vi "Get Variables.vi"(8 "error in (no error)":errorcluster, 11 "functionbase in":refnum<class "functionbase.lvclass">) -> (0 "error out":errorcluster, 2 "Variables":variant, 3 "functionbase out":refnum<class "functionbase.lvclass">)   [LabVIEW 2019, in "LSL.lvlib" / "functionbase.lvclass"]
uses:
  functionbase.lvclass
  typedefs/Variables.ctl
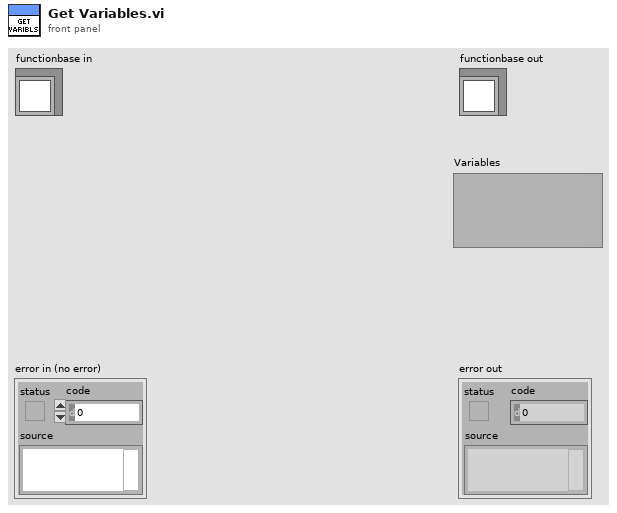
[diagram p1: front panel]
types:
  T1 = typedef "LSL.lvlib/functionbase.lvclass/Variables.ctl" = cluster{"BoringEngineer":string}
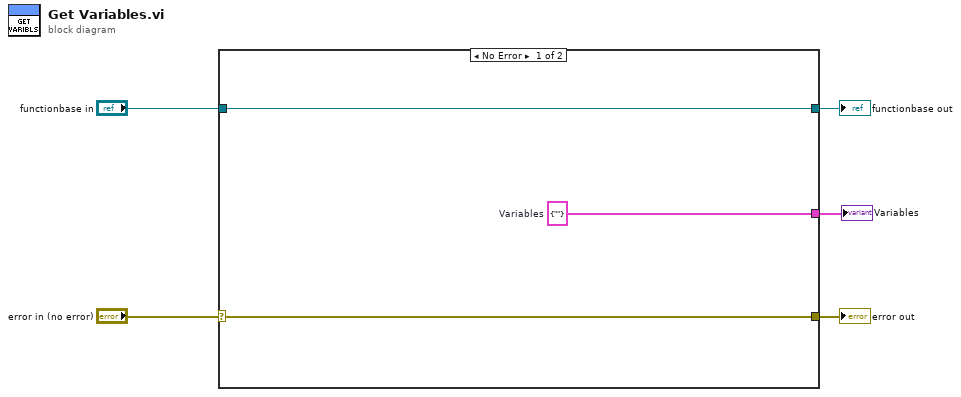
[diagram p0: block diagram]
diagram:
  n1 = case shown="No Error" "error in (no error)" {
    selector: "error in (no error)" -> [w8 w10]
    tunnel: [w8 w10] -> w4
    tunnel: [w7 w9] -> w2
    tunnel: "functionbase in" -> [w7 w9]
    tunnel: [w6 _] -> w1
    frame No Error {
      w6 = T1 {"BoringEngineer"=""}  # Variables
    }
    frame Error {
    }
  }
  "error out" <- w4
  "functionbase out" <- w2
  "Variables" <- w1
